vi "rgsh.vi"(0 "x0":bool, 1 "x1":bool, 3 "x4":bool, 4 "x2":bool, 5 "x3":bool) -> (2 "?":bool, 6 "?":bool, 7 "dec1":bool, 8 "?":bool, 9 "?":bool, 10 "?":bool, 11 "y6":bool, 12 "dec2":bool, 13 "y5":bool, 14 "y0":bool, 15 "y1":bool, 17 "y2":bool, 18 "y3":bool, 19 "y4":bool)   [LabVIEW 2017]
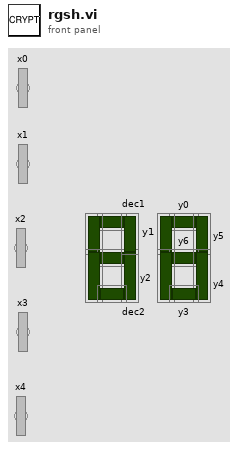
[diagram p1: front panel]
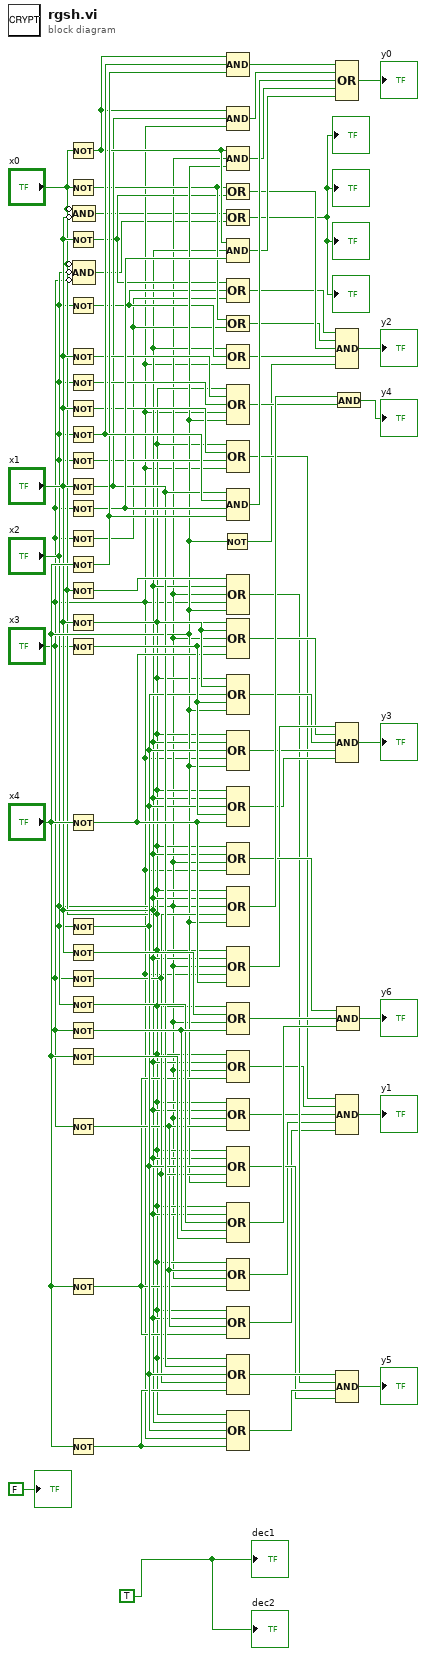
[diagram p0: block diagram]
diagram:
  w1 = TRUE
  n1 = Not(x="x0") -> (.not. x?=w64:bool)
  n2 = Not(x="x0") -> (.not. x?=w17:bool)
  n3 = Not(x="x1") -> (.not. x?=w12:bool)
  n4 = Not(x="x2") -> (.not. x?=w11:bool)
  n5 = Not(x="x1") -> (.not. x?=w62:bool)
  n6 = Not(x="x2") -> (.not. x?=w61:bool)
  n7 = Not(x="x1") -> (.not. x?=w30:bool)
  n8 = Not(x="x2") -> (.not. x?=w66:bool)
  n9 = Not(x="x2") -> (.not. x?=w29:bool)
  n10 = Not(x="x1") -> (.not. x?=w39:bool)
  n11 = Not(x="x3") -> (.not. x?=w63:bool)
  n12 = Not(x="x3") -> (.not. x?=w10:bool)
  n13 = Not(x="x4") -> (.not. x?=w65:bool)
  n14 = Not(x="x0") -> (.not. x?=w40:bool)
  n15 = Not(x="x1") -> (.not. x?=w43:bool)
  n16 = Not(x="x3") -> (.not. x?=w42:bool)
  n17 = Not(x="x4") -> (.not. x?=w41:bool)
  n18 = Not(x="x2") -> (.not. x?=w38:bool)
  n19 = Not(x="x1") -> (.not. x?=w57:bool)
  n20 = Not(x="x3") -> (.not. x?=w37:bool)
  n21 = Not(x="x2") -> (.not. x?=w54:bool)
  n22 = Not(x="x3") -> (.not. x?=w55:bool)
  n23 = Not(x="x4") -> (.not. x?=w56:bool)
  n24 = Not(x="x3") -> (.not. x?=w28:bool)
  n25 = Not(x="x4") -> (.not. x?=w27:bool)
  n26 = Not(x="x4") -> (.not. x?=w36:bool)
  n27 = Compound Arithmetic op=AND(invert "x0", invert "x1") -> (w5:bool)
  n28 = Compound Arithmetic op=AND(invert "x0", invert "x2", invert "x3") -> (w4:bool)
  n29 = Not(x="x4") -> (.not. x?=w18:bool)
  n30 = Compound Arithmetic op=AND(w64, w66, w65) -> (w72:bool)
  n31 = Compound Arithmetic op=AND(w64, w39, "x3") -> (w71:bool)
  n32 = Compound Arithmetic op=AND(w64, "x2", "x4") -> (w69:bool)
  n33 = Compound Arithmetic op=OR(w17, w12) -> (w15:bool)
  n34 = Compound Arithmetic op=OR(w5, w4) -> (→"?" →"?" →"?" →"?":bool)
  n35 = Compound Arithmetic op=AND(w64, "x1", w63) -> (w68:bool)
  n36 = Compound Arithmetic op=OR(w12, w11, w10) -> (w13:bool)
  n37 = Compound Arithmetic op=OR(w17, w10) -> (w14:bool)
  n38 = Compound Arithmetic op=OR("x1", w11, "x3") -> (w16:bool)
  n39 = Compound Arithmetic op=OR("x0", w62, w61, "x3", "x4") -> (w59:bool)
  n40 = Compound Arithmetic op=OR("x0", w30, w29, "x3") -> (w26:bool)
  n41 = Compound Arithmetic op=AND(w39, w66, w63, w65) -> (w70:bool)
  n42 = Compound Arithmetic op=OR(w40, "x1", "x2", "x3", "x4") -> (w34:bool)
  n43 = Compound Arithmetic op=OR("x0", w43, "x2", w42, w41) -> (w48:bool)
  n44 = Compound Arithmetic op=OR("x0", w43, w38, w42, "x4") -> (w47:bool)
  n45 = Compound Arithmetic op=OR("x0", "x1", w38, "x3", "x4") -> (w46:bool)
  n46 = Compound Arithmetic op=OR("x0", "x1", w38, w42, w41) -> (w45:bool)
  n47 = Compound Arithmetic op=OR("x0", "x1", "x2", "x3") -> (w53:bool)
  n48 = Compound Arithmetic op=OR("x0", "x1", "x2", w37, "x4") -> (w60:bool)
  n49 = Compound Arithmetic op=OR("x0", "x1", "x2", "x3", w41) -> (w49:bool)
  n50 = Compound Arithmetic op=OR("x0", w57, "x2", w55) -> (w52:bool)
  n51 = Compound Arithmetic op=OR("x0", "x1", "x2", w27) -> (w25:bool)
  n52 = Compound Arithmetic op=OR("x0", "x1", "x2", w28) -> (w24:bool)
  n53 = Compound Arithmetic op=OR("x0", "x1", w38, w37, "x4") -> (w32:bool)
  n54 = Compound Arithmetic op=OR("x0", "x1", w54, w55, w56) -> (w51:bool)
  n55 = Compound Arithmetic op=OR("x0", w28, "x2", w27) -> (w23:bool)
  n56 = Compound Arithmetic op=OR("x0", "x1", w28, w27) -> (w22:bool)
  n57 = Compound Arithmetic op=OR("x0", w39, w38, w37, w36) -> (w35:bool)
  n58 = Compound Arithmetic op=OR("x0", "x1", w38, "x3", w36) -> (w33:bool)
  n59 = And(x=w60, y=w59) -> (x .and. y?=→"y4":bool)
  n60 = Compound Arithmetic op=OR(w72, w71, w70, w69, w68) -> (→"y0":bool)
  n61 = Compound Arithmetic op=AND(w13, w14, w15, w16, w18) -> (→"y2":bool)
  n62 = Compound Arithmetic op=AND(w49, w48, w47, w46, w45) -> (→"y3":bool)
  n63 = Compound Arithmetic op=AND(w26, w25, w24, w23, w22) -> (→"y1":bool)
  n64 = Compound Arithmetic op=AND(w35, w34, w33, w32) -> (→"y5":bool)
  n65 = Compound Arithmetic op=AND(w53, w52, w51) -> (→"y6":bool)
  "?" <- FALSE
  "dec2" <- w1
  "dec1" <- w1
